vi "GetProcessModeParams.vi"(8 "error in (no error)":errorcluster, 10 "ModeName":string, 11 "TopLevel in":refnum<class "TopLevel.lvclass">) -> (0 "error out":errorcluster, 2 "ProcessModeValues":T1, 3 "TopLevel out":refnum<class "TopLevel.lvclass">)   [LabVIEW 2022 SP3, in "TopLevel.lvclass"]
uses:
  TopLevel.lvclass
  Typedefs/ProcessMode--Cluster.ctl
  Typedefs/processMode--enum.ctl
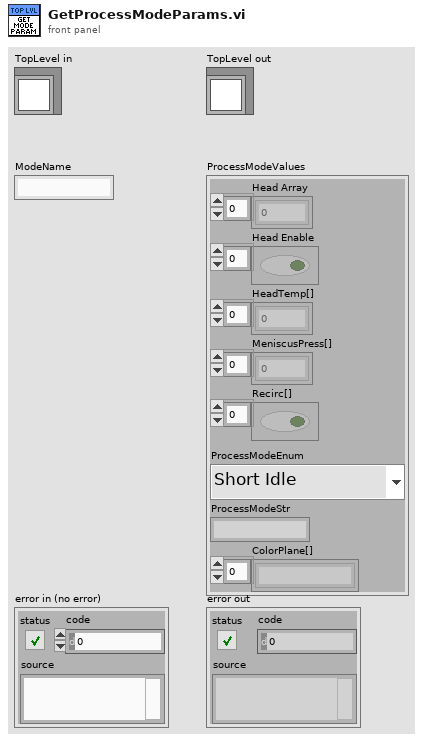
[diagram p1: front panel]
types:
  T1 = typedef "ProcessMode--Cluster.ctl" = cluster{"Head Array":u8[], "Head Enable":bool[], "HeadTemp[]":dbl[], "MeniscusPress[]":dbl[], "Recirc[]":bool[], "ProcessModeEnum":T2, "ProcessModeStr":string, "ColorPlane[]":string[]}
  T2 = typedef "processMode--enum.ctl" = enum16{"Short Idle", "Long Idle ", "C30_Process", "S30_Process"}
  T3 = typedef "DLPConfig_Initialization.ctl" = cluster{"PrinterInitialization":cluster{"Printer":cluster{"#attributes":cluster{"Name":string}}, "VacPumpSet":cluster{"#attributes":cluster{"VacPumpEnable":bool, "VacPumpSpeed":dbl}}, "HIBEnable":cluster{"#attributes":cluster{"HIB1Enable":bool, "HIB2Enable":bool, "HIB3Enable":bool, "HIB4Enable":bool, "HIB5Enable":bool, "HIB6Enable":bool}}, "PrinterCompensation":T4}, "HeadSet":cluster{"HeadProperties":T5[]}, "InkSet":cluster{"Ink":T7[]}, "Troubleshooting":cluster{"PMBLogging":cluster{"#attributes":cluster{"PMBMonitorDuringPrint":bool, "PMBMonitorDuringIdle":bool, "LogSwatheInputData":bool, "LogSwatheOutputData":bool, "LogPrintheadColourPlanes":bool, "LogPMBCommunication":bool, "LogSimulatedOutput":bool, "LogAllPMBCommunicationData":bool, "LogPMBSpace":bool, "ExtendedPMBSpaceLogging":bool, "LogPMBWriteSpeed":bool, "LogUsbRetries":bool}}, "HIBLogging":cluster{"#attributes":cluster{"HIBMonitoringDuringPrint":bool, "HIBMonitoringLog":bool}}}}
  T4 = typedef "DLP2_PrinterCompensationProperties.ctl" = cluster{"#attributes":cluster{"AppName":string, "PrintWeightMultiplier":dbl, "Rotation":bool, "Driver":string, "Server":string, "Database":string, "User":string, "Password":string}}
  T5 = typedef "DLP2_PrinterHeadProperties.ctl" = cluster{"#attributes":T6}
  T6 = typedef "DLPConfig)Init_HeadPropertyAttr--Cluster.ctl" = cluster{"HeadNumber":u8, "Material":string, "HeadLocalX":dbl, "HeadLocalY":dbl, "HeadRotationAngle":dbl, "VH2L_Hi":dbl, "VH2R_Hi":dbl, "VH1LA_Hi":dbl, "VH1LB_Hi":dbl, "VH1RA_Hi":dbl, "VH1RB_Hi":dbl, "VH2L_Lo":dbl, "VH2R_Lo":dbl, "VH1LA_Lo":dbl, "VH1LB_Lo":dbl, "VH1RA_Lo":dbl, "VH1RB_Lo":dbl}
  T7 = typedef "DLP2_PrinterMaterialProperties.ctl" = cluster{"#attributes":cluster{"InkType":string, "PrePrintPurge":bool, "PurgeTime":dbl, "PurgeCount":i32, "Density":dbl, "NumberofDrops":i32, "PrintWeight":dbl, "PrintheadPrime":bool}, "Idle":T8, "Process":T9}
  T8 = typedef "InkIdleNodeConfigXML--Cluster.ctl" = cluster{"ShortIdle":cluster{"#attributes":cluster{"Heat":dbl, "Meniscus":dbl, "Recirculation":bool}}, "LongIdle":cluster{"#attributes":cluster{"Heat":dbl, "Meniscus":dbl, "Recirculation":bool}}}
  T9 = typedef "InkProcessNodeConfigXML--Cluster.ctl" = cluster{"C30_Process":cluster{"#attributes":cluster{"Heat":dbl, "Meniscus":dbl, "Recirculation":bool, "ColorPlane":string}}, "S30_Process":cluster{"#attributes":cluster{"Heat":dbl, "Meniscus":dbl, "Recirculation":bool, "ColorPlane":string}}}
  T10 = typedef "TD Dynamic CVT DVR--ref.ctl" = refnum<data-value>
  T11 = cluster{"HIB1Enable":bool, "HIB2Enable":bool, "HIB3Enable":bool, "HIB4Enable":bool, "HIB5Enable":bool, "HIB6Enable":bool}
  T12 = typedef "processMode_parameters--cluster.ctl" = cluster{"Head Array":u8[], "C30ProcessHeat[]":dbl[], "ShortIdleHeat[]":dbl[], "LongIdleHeat[]":dbl[], "C30ProcessMeniscus[]":dbl[], "ShortIdleMeniscus[]":dbl[], "LongIdleMeniscus[]":dbl[], "C30ProcessRecirc[]":bool[], "ShortIdleRecirc[]":bool[], "LongIdleRecirc[]":bool[], "S30ProcessHeat[]":dbl[], "S30ProcessMeniscus[]":dbl[], "S30ProcessRecirc[]":bool[], "C30ProcessColorPlane[]":string[], "S30ProcessColorPlane[]":string[]}
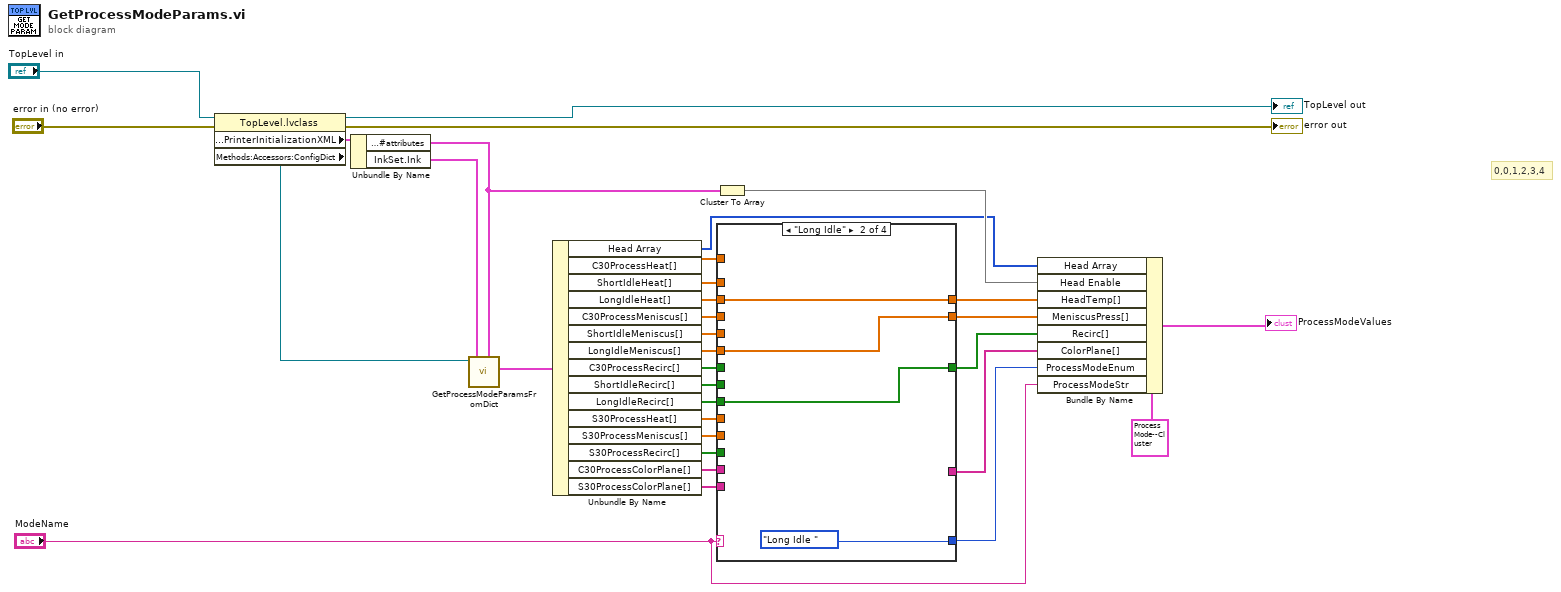
[diagram p0: block diagram]
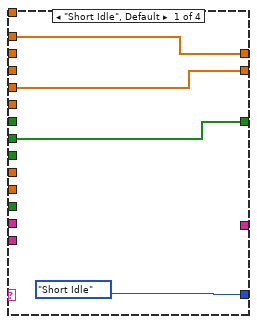
[diagram p2: hidden frame]
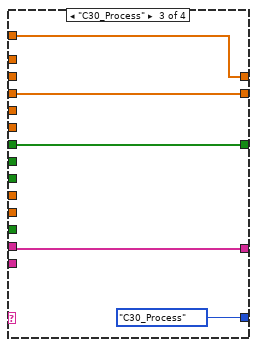
[diagram p3: hidden frame]
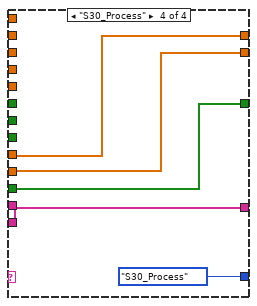
[diagram p4: hidden frame]
diagram:
  # "0,0,1,2,3,4"
  n1 = property class="TopLevel.lvclass"(reference="TopLevel in", error in="error in (no error)") -> (reference out=→"TopLevel out":refnum<class "TopLevel.lvclass">, error out=→"error out":errorcluster, "Methods:Accessors:PrinterInitializationXML"=w8:T3, "Methods:Accessors:ConfigDict"=w11:T10)
  n2 = Unbundle By Name(w8) -> ("PrinterInitialization.HIBEnable.#attributes"=w25:T11, "InkSet.Ink"=w12:T7[])
  n3 = call "GetProcessModeParamsFromDict.vi"("PrinterInitialization.HIBEnable.#attributes"=w25, "Ink"=w12, "Data Value Reference in"=w11) -> ("ProcessModeParams"=w13:T12)  [unwired: 8 in]
  n4 = Unbundle By Name(w13) -> ("Head Array"=w29:u8[], "C30ProcessHeat[]"=w14:dbl[], "ShortIdleHeat[]"=w15:dbl[], "LongIdleHeat[]"=w16:dbl[], "C30ProcessMeniscus[]"=w17:dbl[], "ShortIdleMeniscus[]"=w18:dbl[], "LongIdleMeniscus[]"=w19:dbl[], "C30ProcessRecirc[]"=w20:bool[], "ShortIdleRecirc[]"=w21:bool[], "LongIdleRecirc[]"=w22:bool[], "S30ProcessHeat[]"=w6:dbl[], "S30ProcessMeniscus[]"=w5:dbl[], "S30ProcessRecirc[]"=w4:bool[], "C30ProcessColorPlane[]"=w3:string[], "S30ProcessColorPlane[]"=w2:string[])
  n5 = Cluster To Array(cluster=w25) -> (array=w30:bool[])
  n6 = case shown="\"Long Idle\"" "ModeName" {
    tunnel: w16 -> [_ w41 _ _]
    tunnel: w15 -> [w37 _ _ _]
    tunnel: w14 -> [_ _ w46 _]
    tunnel: [w37 w41 w46 w48] -> w31
    tunnel: [processMode--enum."Short Idle" ("ProcessMode") processMode--enum."Long Idle " ("ProcessMode") processMode--enum."C30_Process" ("ProcessMode") processMode--enum."S30_Process" ("ProcessMode")] -> w27
    tunnel: w17 -> [_ _ w44 _]
    tunnel: w18 -> [w35 _ _ _]
    tunnel: w19 -> [_ w39 _ _]
    tunnel: w20 -> [_ _ w43 _]
    tunnel: w21 -> [w34 _ _ _]
    tunnel: w22 -> [_ w38 _ _]
    tunnel: [w35 w39 w44 w49] -> w32
    tunnel: [w34 w38 w43 w50] -> w33
    tunnel: w6 -> [_ _ _ w48]
    tunnel: w5 -> [_ _ _ w49]
    tunnel: w4 -> [_ _ _ w50]
    tunnel: w3 -> [_ _ w42 _]
    tunnel: w2 -> [_ _ _ w47]
    tunnel: [_ _ w42 w47] -> w1
    frame "Short Idle", Default {
    }
    frame "Long Idle" {
    }
    frame "C30_Process" {
    }
    frame "S30_Process" {
    }
  }
  n7 = Bundle By Name(cluster=T1 {"Head Array"=[], "Head Enable"=[], "HeadTemp[]"=[], "MeniscusPress[]"=[], "Recirc[]"=[], "ProcessModeEnum"=enum."Long Idle ", "ProcessModeStr"="", "ColorPlane[]"=[]} ("ProcessModeValues"), "Head Array"=w29, "Head Enable"=w30, "HeadTemp[]"=w31, "MeniscusPress[]"=w32, "Recirc[]"=w33, "ColorPlane[]"=w1, "ProcessModeEnum"=w27, "ProcessModeStr"="ModeName") -> (→"ProcessModeValues":T1)
